vi "task.directory_lua.vi"(5 "LuaVIEW reference":T1) -> (15 "error out":errorcluster)   [LabVIEW 2012]
doc: "Return the path to the directory in which the task's main script resides.\nResults:\nstr:directory\nErrors:\nFunction must be called from a task context but was not.\nTask script was provided as a string and not a file.\nTask script does not reside on a local filesystem."
uses:
  typedefs/t_LuaVIEW Reference.ctl
  subvis/private/LuaVIEW Push (path).vi
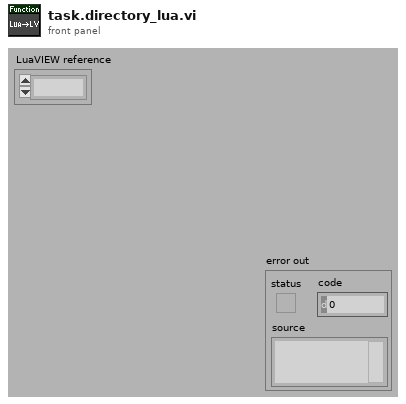
[diagram p1: front panel]
types:
  T1 = typedef "t_LuaVIEW Reference.ctl" = refnum<k1>
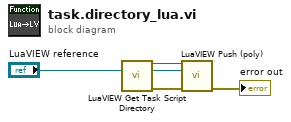
[diagram p0: block diagram]
diagram:
  n1 = call "LuaVIEW Get Task Script Directory.vi"("LuaVIEW reference in"="LuaVIEW reference") -> ("task script directory"=w1:path, "LuaVIEW reference out"=w2:T1, "error out"=w4:errorcluster)  [unwired: 12 in]
  n2 = call-poly "LuaVIEW Push (poly).vi"("path"=w1, "LuaVIEW reference in"=w2, "error in (no error)"=w4) -> ("error out"=→"error out":errorcluster)  [unwired: 11 in, 1 out]
